vi "Build.vi"(8 "error in (no error)":errorcluster, 11 "Composed Column Factory in":refnum<class "Composed Column Factory.lvclass">) -> (0 "error out":errorcluster, 2 "Column":refnum<class "Column Interface.lvclass">, 3 "Composed Column Factory out":refnum<class "Composed Column Factory.lvclass">)   [LabVIEW 2020, in "Composed Columns.lvlib" / "Composed Column Factory.lvclass"]
uses:
  Composed Column Factory.lvclass
  Column Interface/Column Interface Class/Column Interface.lvclass
  Composed Column Factory.lvclass/Composed Column Factory.ctl
  Column/Composed Column.lvclass
  C:/Users/User/Desktop/Raman Program/Database OOP/source/Database OOP/Column Libraries/Column Interface/Column Interface Class/Column Interface.lvclass
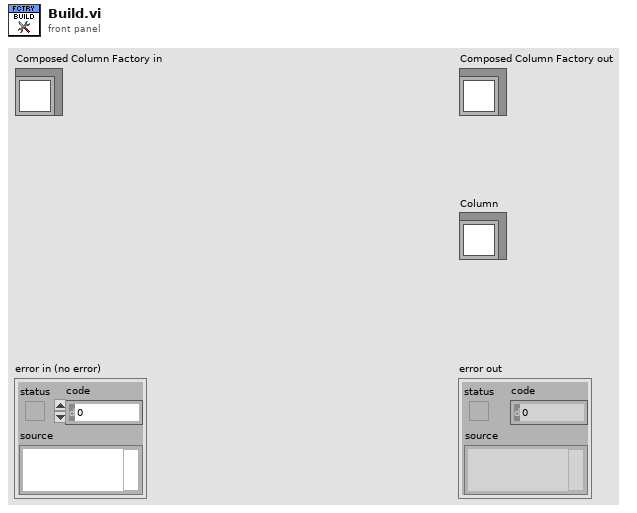
[diagram p1: front panel]
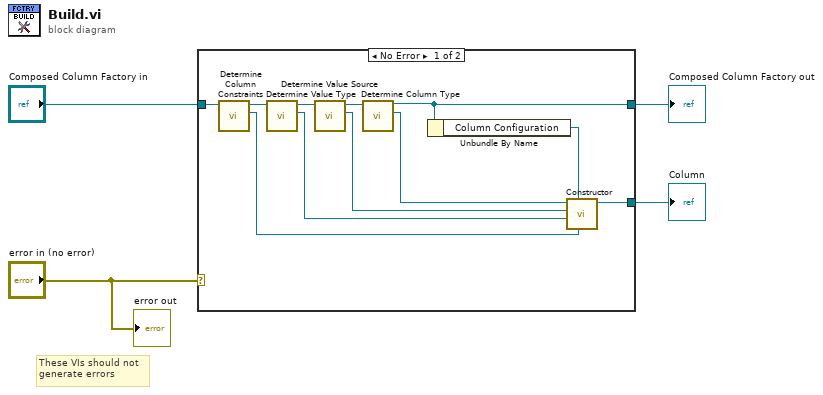
[diagram p0: block diagram]
diagram:
  # "These VIs should not\ngenerate errors"
  n1 = case shown="No Error" "error in (no error)" {
    tunnel: "Composed Column Factory in" -> [w13 w16]
    tunnel: [w5 w16] -> w3
    tunnel: [w15 _] -> w2
    frame No Error {
      n2 = call-dynamic "Determine Column Constraints.vi"("Composed Column Factory in"=w13) -> ("Column Constraints"=w12:refnum<class "Constraint Manager.lvclass">, "Composed Column Factory out"=w11:refnum<class "Composed Column Factory.lvclass">)  [unwired: 8 in, 1 out]
      n3 = call-dynamic "Determine Value Type.vi"("Composed Column Factory in"=w11) -> ("Value Type"=w10:refnum<class "Value Type.lvclass">, "Composed Column Factory out"=w7:refnum<class "Composed Column Factory.lvclass">)  [unwired: 8 in, 1 out]
      n4 = call-dynamic "Determine Value Source.vi"("Composed Column Factory in"=w7) -> ("Value Source"=w9:refnum<class "Value Source.lvclass">, "Composed Column Factory out"=w6:refnum<class "Composed Column Factory.lvclass">)  [unwired: 8 in, 1 out]
      n5 = call-dynamic "Determine Column Type.vi"("Composed Column Factory in"=w6) -> ("Column"=w8:refnum<class "Composed Column.lvclass">, "Composed Column Factory out"=w5:refnum<class "Composed Column Factory.lvclass">)  [unwired: 8 in, 1 out]
      n6 = Unbundle By Name(w5) -> ("Column Configuration"=w14:refnum<class "Column Configuration.lvclass">)
      n7 = call "Constructor.vi"("Check Manager"=w12, "Configuration"=w14, "Value Type"=w10, "Value Source"=w9, "Composed Column in"=w8) -> ("Composed Column out"=w15:refnum<class "Composed Column.lvclass">)  [unwired: 5 in, 1 out]
    }
    frame Error {
    }
  }
  "Composed Column Factory out" <- w3
  "Column" <- w2
  "error out" <- "error in (no error)"
